vi "Evaluate Part 2_debugging.vi"() -> ()   [LabVIEW 2020]
uses:
  Proto/Proto.lvclass
panel:
  out "Array 4":string[](array[string])
  out "Array 3":string[](array[string])
  out "Parsed Array 2":string[](array[string])
  out "Array 2":i32[](array[numeric])
  out "Boolean array":bool[](array[boolean])
  out "x-y":u64
  out "x = y?":bool
  out "number":u64
  out "Array":bool[](array[boolean])
  in  "Input":string="x00: 1\nx01: 0\nx02: 1\nx03: 1\nx04: 0\ny00: 1\ny01: 1\ny02: 1\ny03: 1\ny04: 1\n\nntg XOR fgs -> mjb\ny02 OR x01 -> tnw\nkwq OR kpj -> z05\nx00 OR x03 -> fst\ntgd XOR rvg -> z01\nvdt OR tnw -> bfw\nbfw AND frj -> z10\nffh OR nrd -> bqk\ny00 AND y03 -> djm\ny03 OR y00 -> psh\nbqk OR frj -> z08\ntnw OR fst -> frj\ngnj AND tgd -> z11\nbfw XOR mjb -> z00\nx03 OR x00 -> vdt\ngnj AND wpb -> z02\nx04 AND y00 -> kjc\ndjm OR pbm -> qhw\nnrd AND vdt -> hwm\nkjc AND fst -> rvg\ny04 OR y02 -> fgs\ny01 AND x02 -> pbm\nntg OR kjc -> kwq\npsh XOR fgs -> tgd\nqhw XOR tgd -> z09\npbm OR djm -> kpj\nx03 XOR y03 -> ffh\nx00 XOR y04 -> ntg\nbfw OR bqk -> z06\nnrd XOR fgs -> wpb\nfrj XOR qhw -> z04\nbqk OR frj -> z07\ny03 OR x01 -> nrd\nhwm AND bqk -> z03\ntgd XOR rvg -> z12\ntnw OR pbm -> gnj"
  # "2947015374 too low\n\n282578783305985 too high\n66055249060558"
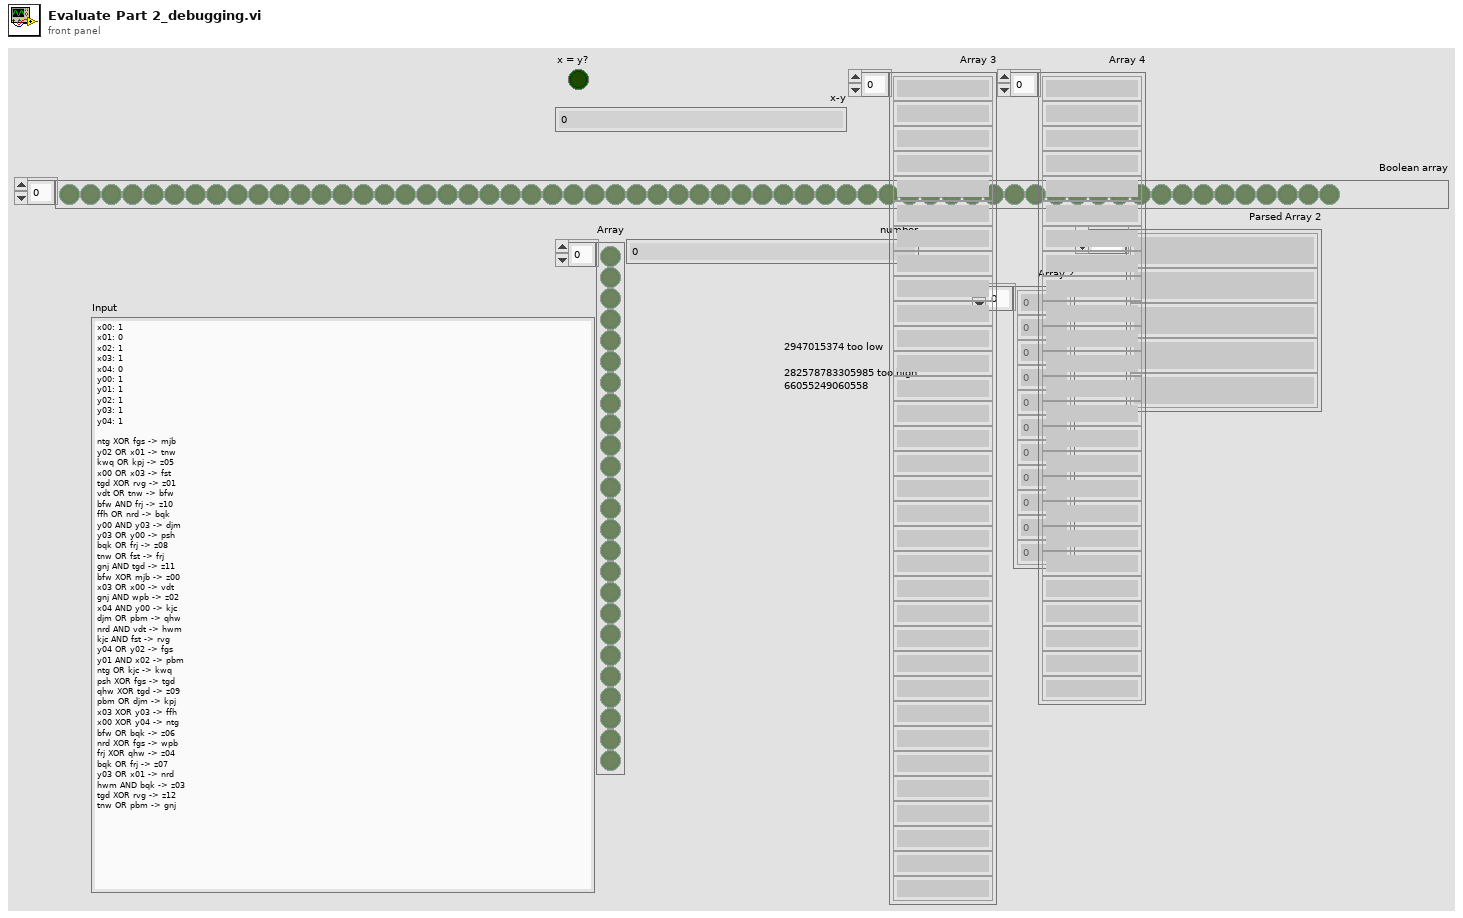
[diagram p1: front panel]
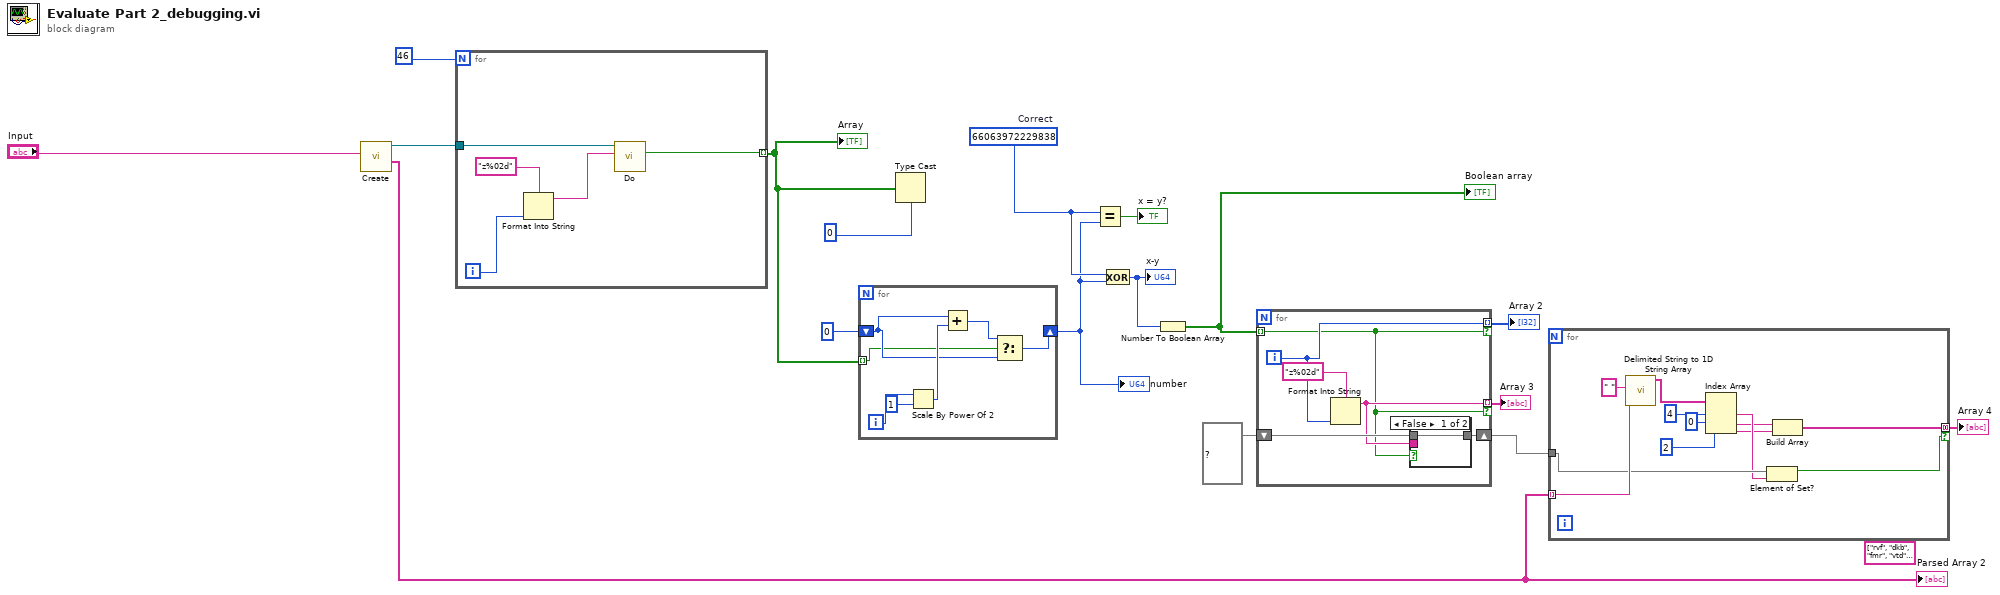
[diagram p0: block diagram]
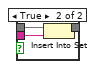
[diagram p2: hidden frame]
diagram:
  (unwired) string[] ["rvf", "dkb", "fmr", "vtd", "y16", "x16", "gdq", "chf", "krw", "vnk", "mvn", "wjt", "dtn", "ntn", "wkw", "jgr", "fcd", "mgc", "pns", "tsc"] ("Array 4")
  w10 = u64 66063972229838  # Correct
  n1 = call "Create.vi"("Input"="Input") -> ("Parsed Array 2"=w2:string[], "Proto"=w16:refnum<class "Proto.lvclass">)  [unwired: 9 in]
  "Parsed Array 2" <- w2
  n2 = for {
    N: 46 -> [_]
    tunnel: w16 -> [w22]
    tunnel: [w18] -> w14 mode=indexing
    i -> [w20]
    n3 = Format Into String(format string="z%02d", w20) -> (resulting string=w19:string)  [unwired: 2 in, 1 out]
    n4 = call "Do.vi"("Key"=w19, "Proto in"=w22) -> ("Value"=w18:bool)  [unwired: 7 in, 2 out]
  }
  "Array" <- w14
  n5 = for {
    tunnel: w14 -> [w25] mode=indexing
    shift-right: [w23] -> w9
    shift-left: u64 0 ("number") -> [w26]
    i -> [w29]
    n6 = Scale By Power Of 2(n=w29, x=u64 1) -> (x*2^n=w27:u64)
    n7 = Add(x=w26, y=w27) -> (x+y=w24:u64)
    n8 = Select(t=w24, s=w25, f=w26) -> (s? t:f=w23:u64)
  }
  "number" <- w9
  n9 = Type Cast(type=u64 0 ("number"), x=w14) -> ()  [unwired: 1 out]
  n10 = Equal?(x=w10, y=w9) -> (x = y?=→"x = y?":bool)
  n11 = Exclusive Or(1:w9, 2:w10) -> (0:w8:u64)
  "x-y" <- w8
  n12 = Number To Boolean Array(number=w8) -> (Boolean array=w7:bool[])
  "Boolean array" <- w7
  n13 = for {
    tunnel: w7 -> [w30] mode=indexing
    tunnel: [w35] -> w6 mode=indexing if=w30
    tunnel: [w32] -> w5 mode=indexing if=w30
    shift-right: [w31] -> w3
    shift-left: set{string} {} ("set in") -> [w33]
    i -> [w35]
    n14 = Format Into String(format string="z%02d", w35) -> (resulting string=w32:string)  [unwired: 2 in, 1 out]
    n15 = case shown="False" w30 {
      tunnel: w33 -> [w36 w39]
      tunnel: w32 -> [_ w38]
      tunnel: [w36 w37] -> w31
      frame False {
      }
      frame True {
        n16 = Insert Into Set(10:w38, 11:w39) -> (3:w37:set{string})  [unwired: 1 out]
      }
    }
  }
  "Array 2" <- w6
  "Array 3" <- w5
  n17 = for {
    tunnel: w3 -> [w47]
    tunnel: w2 -> [w48] mode=indexing
    tunnel: [w41] -> w1 mode=concatenating if=w40
    n18 = call <vilib>:"Delimited String to 1D String Array.vi"("delimiter"=" ", "delimited string"=w48) -> ("string array"=w50:string[])  [unwired: 9 in]
    n19 = Index Array(array=w50, index #1=4 ("index"), index #2=0 ("index"), index #3=2 ("index")) -> (element #1=w46:string, element #2=w42:string, element #3=w43:string)
    n20 = Element of Set?(10:w46, 11:w47) -> (3:w40:bool)
    n21 = Build Array(w42, w43) -> (w41:string[])
  }
  "Array 4" <- w1
